vi "LINC Packet Decode.vi"(7 "little endian":bool, 8 "include unit (F)":bool, 9 "binary value (F)":bool, 10 "item formats":T1[](array[typedef]), 11 "data in":string) -> (2 "decoded items":string[](array[string]))   [LabVIEW 2018, in "STEPkgDriver_LINC.lvlib" / "LINC.lvclass"]
uses:
  LINC.lvclass
  STEPkgDriver_LINC.lvlib
  LINC Format Prototype.ctl
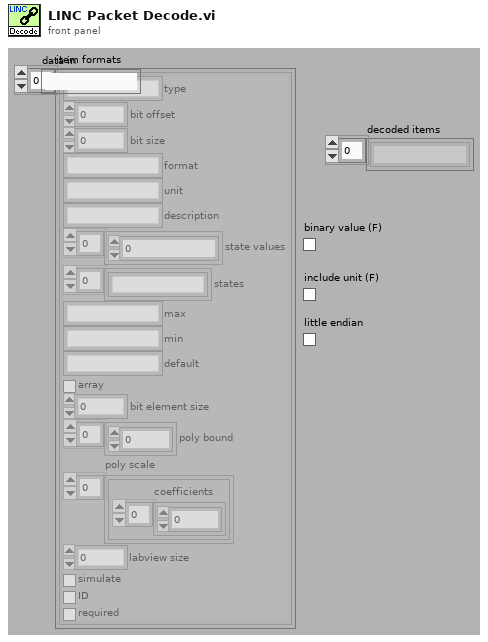
[diagram p1: front panel]
types:
  T1 = typedef "STEPkgDriver_LINC.lvlib/LINC Format Prototype.ctl" = cluster{"type":string, "bit offset":i32, "bit size":i32, "format":string, "unit":string, "description":string, "state values":i64[], "states":string[], "max":string, "min":string, "default":string, "array":bool, "bit element size":i32, "poly bound":dbl[], "poly scale":cluster{"coefficients":dbl[]}[], "labview size":i32, "simulate":bool, "ID":bool, "required":bool}
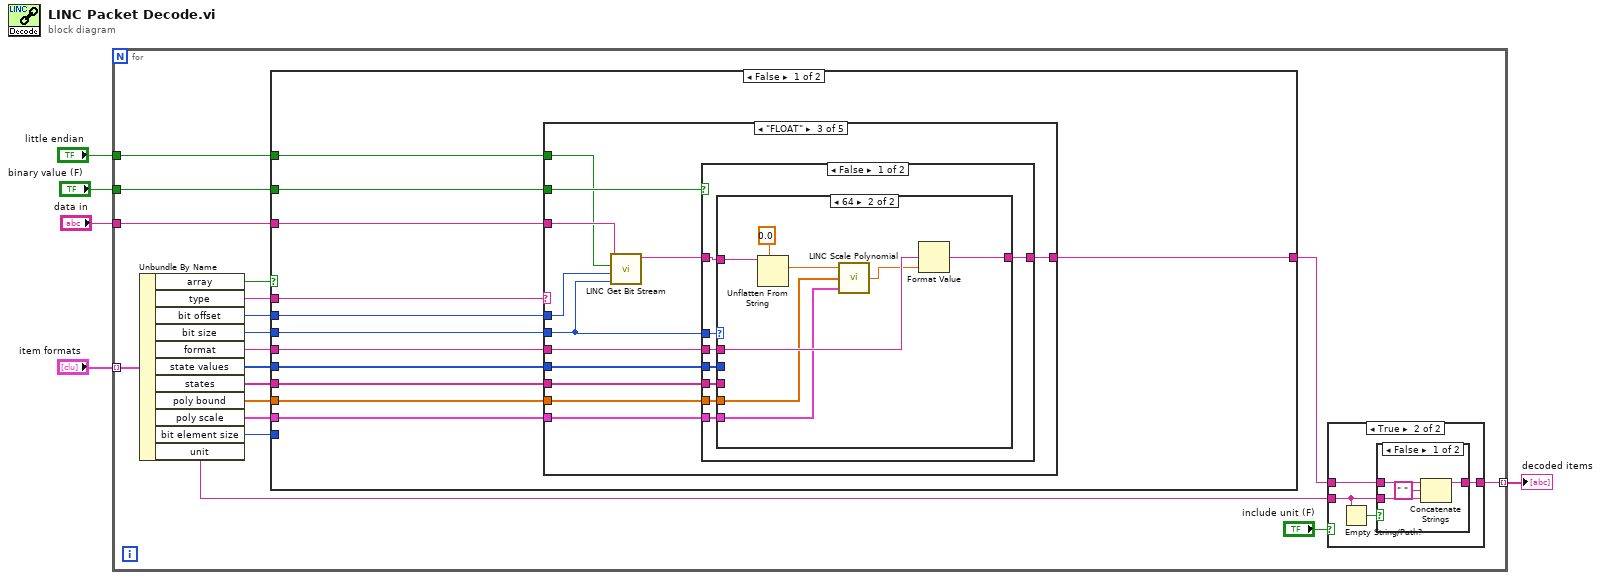
[diagram p0: block diagram]
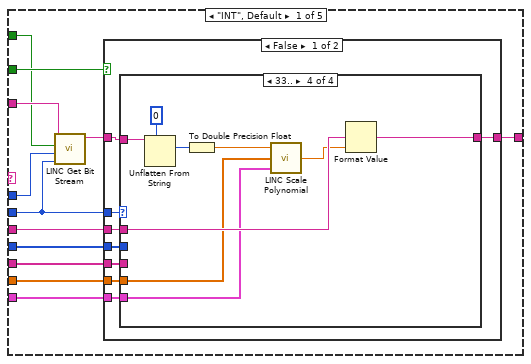
[diagram p2: hidden frame]
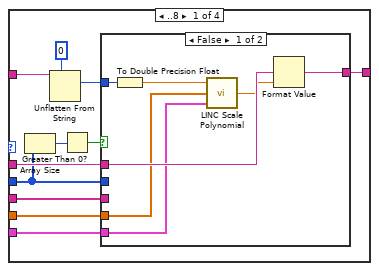
[diagram p3: hidden frame]
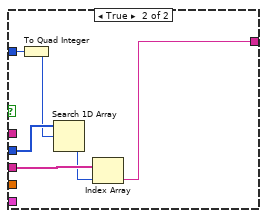
[diagram p4: hidden frame]
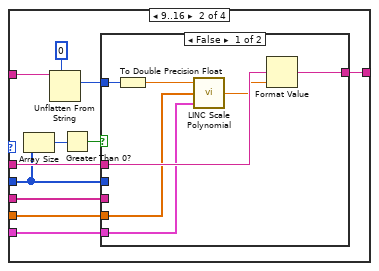
[diagram p5: hidden frame]
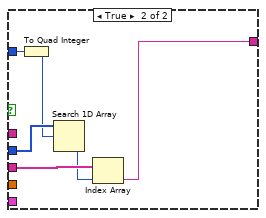
[diagram p6: hidden frame]
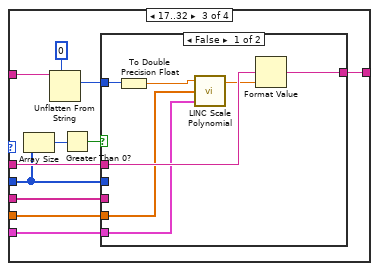
[diagram p7: hidden frame]
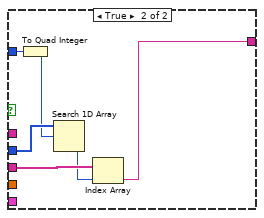
[diagram p8: hidden frame]
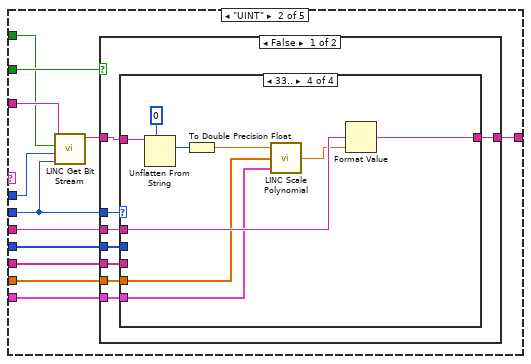
[diagram p10: hidden frame]
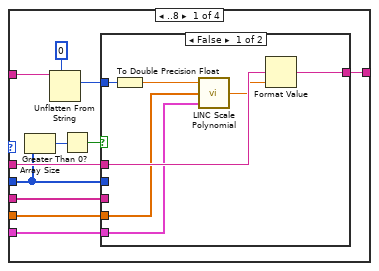
[diagram p11: hidden frame]
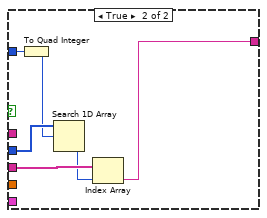
[diagram p12: hidden frame]
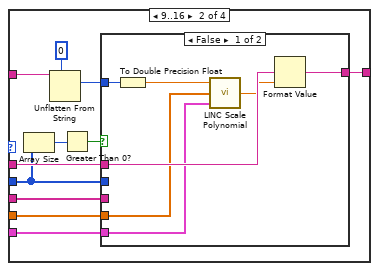
[diagram p13: hidden frame]
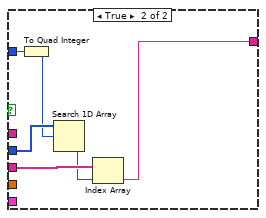
[diagram p14: hidden frame]
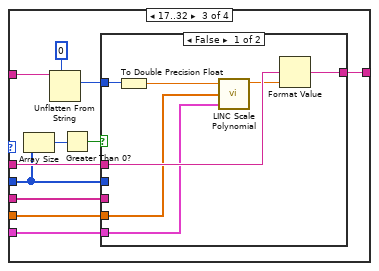
[diagram p15: hidden frame]
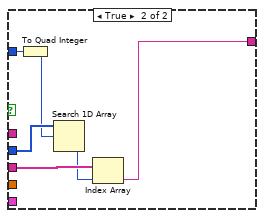
[diagram p16: hidden frame]
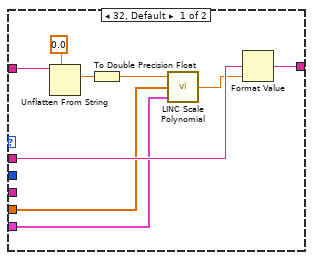
[diagram p18: hidden frame]
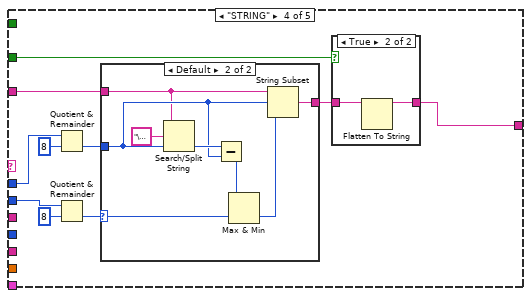
[diagram p20: hidden frame]
diagram:
  n1 = for {
    tunnel: "data in" -> [w13]
    tunnel: "item formats" -> [w23] mode=indexing
    tunnel: [w17] -> w5 mode=indexing
    tunnel: "binary value (F)" -> [w9]
    tunnel: "little endian" -> [w8]
    n2 = Unbundle By Name(w23) -> ("array"=w7:bool, "type"=w22:string, "bit offset"=w14:i32, "bit size"=w15:i32, "format"=w21:string, "state values"=w18:i64[], "states"=w20:string[], "poly bound"=w12:dbl[], "poly scale"=w6:cluster{"coefficients":dbl[]}[], "bit element size"=w16:i32, "unit"=w19:string)
    n3 = case shown="False" w7 {
      tunnel: w22 -> [w35 w342]
      tunnel: w15 -> [w30 w333]
      tunnel: w21 -> [w34 w345]
      tunnel: w20 -> [w33 w343]
      tunnel: [w32 w346] -> w11
      tunnel: w18 -> [w31 w344]
      tunnel: w16 -> [_ w339]
      tunnel: w14 -> [w27 w334]
      tunnel: w12 -> [w29 _]
      tunnel: w13 -> [w28 w335]
      tunnel: w9 -> [w26 w330]
      tunnel: w8 -> [w25 w329]
      tunnel: w6 -> [w24 _]
      frame False {
        n4 = case shown="\"FLOAT\"" w35 {
          tunnel: w30 -> [w43 w141 w241 w282 w306]
          tunnel: [w45 w147 w249 w279 w303] -> w32
          tunnel: w34 -> [w42 w149 w251 _ _]
          tunnel: w33 -> [w40 w148 w250 _ _]
          tunnel: w31 -> [w41 w146 w248 _ _]
          tunnel: w29 -> [w39 w145 w247 _ _]
          tunnel: w28 -> [w47 w144 w245 w284 w308]
          tunnel: w27 -> [w46 w142 w242 w283 w307]
          tunnel: w26 -> [w38 w140 w246 w281 w305]
          tunnel: w25 -> [w37 w139 w243 _ _]
          tunnel: w24 -> [w36 w138 w240 _ _]
          frame "INT", Default {
            n5 = call "LINC Get Bit Stream.vi"("bit size"=w43, "bit offset"=w46, "little endian"=w37, "data in"=w47) -> ("data out"=w44:string)  [unwired: 6 in, 1 out]
            n6 = case shown="False" w38 {
              tunnel: [w55 w137] -> w45
              tunnel: w44 -> [w54 w137]
              tunnel: w43 -> [w53 _]
              tunnel: w42 -> [w52 _]
              tunnel: w41 -> [w51 _]
              tunnel: w40 -> [w50 _]
              tunnel: w39 -> [w49 _]
              tunnel: w36 -> [w48 _]
              frame False {
                n7 = case shown="33.." w53 {
                  tunnel: w54 -> [w66 w90 w114 w136]
                  tunnel: w52 -> [w61 w85 w109 w134]
                  tunnel: w50 -> [w62 w86 w110 _]
                  tunnel: [w59 w83 w107 w133] -> w55
                  tunnel: w51 -> [w58 w82 w106 _]
                  tunnel: w49 -> [w57 w81 w105 w129]
                  tunnel: w48 -> [w56 w80 w104 w128]
                  frame ..8 {
                    n8 = Array Size(array=w58) -> (size(s)=w64:i32)
                    n9 = Unflatten From String(type=i8 0, binary string=w66) -> (value=w60:i8)  [unwired: 3 in, 2 out]
                    n10 = Greater Than 0?(x=w64) -> (x > 0?=w63:bool)
                    n11 = case shown="False" w63 {
                      tunnel: w62 -> [_ w76]
                      tunnel: w61 -> [w73 _]
                      tunnel: w60 -> [w70 w79]
                      tunnel: [w72 w74] -> w59
                      tunnel: w58 -> [_ w78]
                      tunnel: w57 -> [w68 _]
                      tunnel: w56 -> [w67 _]
                      frame False {
                        n12 = To Double Precision Float(number=w70) -> (double precision float=w71:dbl)
                        n13 = call "LINC Scale Polynomial.vi"("poly scale"=w67, "poly bounds"=w68, "unscaled value"=w71) -> ("scaled value"=w69:dbl)
                        n14 = Format Value(format string=w73, value (0)=w69) -> (output string=w72:string)  [unwired: 1 in]
                      }
                      frame True {
                        n15 = To Quad Integer(1:w79) -> (0:w77:i64)
                        n16 = Search 1D Array(1D array=w78, element=w77) -> (index of element=w75:i32)  [unwired: 1 in]
                        n17 = Index Array(array=w76, index=w75) -> (element=w74:string)
                      }
                    }
                  }
                  frame 9..16 {
                    n18 = Array Size(array=w82) -> (size(s)=w88:i32)
                    n19 = Unflatten From String(type=i16 0, binary string=w90) -> (value=w84:i16)  [unwired: 3 in, 2 out]
                    n20 = Greater Than 0?(x=w88) -> (x > 0?=w87:bool)
                    n21 = case shown="False" w87 {
                      tunnel: w86 -> [_ w100]
                      tunnel: w85 -> [w97 _]
                      tunnel: w84 -> [w94 w103]
                      tunnel: [w96 w98] -> w83
                      tunnel: w82 -> [_ w102]
                      tunnel: w81 -> [w92 _]
                      tunnel: w80 -> [w91 _]
                      frame False {
                        n22 = To Double Precision Float(number=w94) -> (double precision float=w95:dbl)
                        n23 = call "LINC Scale Polynomial.vi"("poly scale"=w91, "poly bounds"=w92, "unscaled value"=w95) -> ("scaled value"=w93:dbl)
                        n24 = Format Value(format string=w97, value (0)=w93) -> (output string=w96:string)  [unwired: 1 in]
                      }
                      frame True {
                        n25 = To Quad Integer(1:w103) -> (0:w101:i64)
                        n26 = Search 1D Array(1D array=w102, element=w101) -> (index of element=w99:i32)  [unwired: 1 in]
                        n27 = Index Array(array=w100, index=w99) -> (element=w98:string)
                      }
                    }
                  }
                  frame 17..32 {
                    n28 = Array Size(array=w106) -> (size(s)=w112:i32)
                    n29 = Unflatten From String(type=0, binary string=w114) -> (value=w108:i32)  [unwired: 3 in, 2 out]
                    n30 = Greater Than 0?(x=w112) -> (x > 0?=w111:bool)
                    n31 = case shown="False" w111 {
                      tunnel: w110 -> [_ w124]
                      tunnel: w109 -> [w121 _]
                      tunnel: w108 -> [w118 w127]
                      tunnel: [w120 w122] -> w107
                      tunnel: w106 -> [_ w126]
                      tunnel: w105 -> [w116 _]
                      tunnel: w104 -> [w115 _]
                      frame False {
                        n32 = To Double Precision Float(number=w118) -> (double precision float=w119:dbl)
                        n33 = call "LINC Scale Polynomial.vi"("poly scale"=w115, "poly bounds"=w116, "unscaled value"=w119) -> ("scaled value"=w117:dbl)
                        n34 = Format Value(format string=w121, value (0)=w117) -> (output string=w120:string)  [unwired: 1 in]
                      }
                      frame True {
                        n35 = To Quad Integer(1:w127) -> (0:w125:i64)
                        n36 = Search 1D Array(1D array=w126, element=w125) -> (index of element=w123:i32)  [unwired: 1 in]
                        n37 = Index Array(array=w124, index=w123) -> (element=w122:string)
                      }
                    }
                  }
                  frame 33.. {
                    n38 = Unflatten From String(type=i64 0, binary string=w136) -> (value=w131:i64)  [unwired: 3 in, 2 out]
                    n39 = To Double Precision Float(number=w131) -> (double precision float=w132:dbl)
                    n40 = call "LINC Scale Polynomial.vi"("poly scale"=w128, "poly bounds"=w129, "unscaled value"=w132) -> ("scaled value"=w130:dbl)
                    n41 = Format Value(format string=w134, value (0)=w130) -> (output string=w133:string)  [unwired: 1 in]
                  }
                }
              }
              frame True {
              }
            }
          }
          frame "UINT" {
            n42 = call "LINC Get Bit Stream.vi"("bit size"=w141, "bit offset"=w142, "little endian"=w139, "data in"=w144) -> ("data out"=w143:string)  [unwired: 6 in, 1 out]
            n43 = case shown="False" w140 {
              tunnel: w149 -> [w157 _]
              tunnel: w148 -> [w156 _]
              tunnel: [w155 w239] -> w147
              tunnel: w146 -> [w154 _]
              tunnel: w145 -> [w153 _]
              tunnel: w143 -> [w152 w239]
              tunnel: w141 -> [w151 _]
              tunnel: w138 -> [w150 _]
              frame False {
                n44 = case shown="33.." w151 {
                  tunnel: w152 -> [w168 w192 w216 w238]
                  tunnel: w157 -> [w163 w187 w211 w236]
                  tunnel: w156 -> [w164 w188 w212 _]
                  tunnel: [w161 w185 w209 w235] -> w155
                  tunnel: w154 -> [w160 w184 w208 _]
                  tunnel: w153 -> [w159 w183 w207 w231]
                  tunnel: w150 -> [w158 w182 w206 w230]
                  frame ..8 {
                    n45 = Array Size(array=w160) -> (size(s)=w166:i32)
                    n46 = Unflatten From String(type=u8 0, binary string=w168) -> (value=w162:u8)  [unwired: 3 in, 2 out]
                    n47 = Greater Than 0?(x=w166) -> (x > 0?=w165:bool)
                    n48 = case shown="False" w165 {
                      tunnel: w164 -> [_ w178]
                      tunnel: w163 -> [w175 _]
                      tunnel: w162 -> [w172 w181]
                      tunnel: [w174 w176] -> w161
                      tunnel: w160 -> [_ w180]
                      tunnel: w159 -> [w170 _]
                      tunnel: w158 -> [w169 _]
                      frame False {
                        n49 = To Double Precision Float(number=w172) -> (double precision float=w173:dbl)
                        n50 = call "LINC Scale Polynomial.vi"("poly scale"=w169, "poly bounds"=w170, "unscaled value"=w173) -> ("scaled value"=w171:dbl)
                        n51 = Format Value(format string=w175, value (0)=w171) -> (output string=w174:string)  [unwired: 1 in]
                      }
                      frame True {
                        n52 = To Quad Integer(1:w181) -> (0:w179:i64)
                        n53 = Search 1D Array(1D array=w180, element=w179) -> (index of element=w177:i32)  [unwired: 1 in]
                        n54 = Index Array(array=w178, index=w177) -> (element=w176:string)
                      }
                    }
                  }
                  frame 9..16 {
                    n55 = Array Size(array=w184) -> (size(s)=w190:i32)
                    n56 = Unflatten From String(type=u16 0, binary string=w192) -> (value=w186:u16)  [unwired: 3 in, 2 out]
                    n57 = Greater Than 0?(x=w190) -> (x > 0?=w189:bool)
                    n58 = case shown="False" w189 {
                      tunnel: w188 -> [_ w202]
                      tunnel: w187 -> [w199 _]
                      tunnel: w186 -> [w196 w205]
                      tunnel: [w198 w200] -> w185
                      tunnel: w184 -> [_ w204]
                      tunnel: w183 -> [w194 _]
                      tunnel: w182 -> [w193 _]
                      frame False {
                        n59 = To Double Precision Float(number=w196) -> (double precision float=w197:dbl)
                        n60 = call "LINC Scale Polynomial.vi"("poly scale"=w193, "poly bounds"=w194, "unscaled value"=w197) -> ("scaled value"=w195:dbl)
                        n61 = Format Value(format string=w199, value (0)=w195) -> (output string=w198:string)  [unwired: 1 in]
                      }
                      frame True {
                        n62 = To Quad Integer(1:w205) -> (0:w203:i64)
                        n63 = Search 1D Array(1D array=w204, element=w203) -> (index of element=w201:i32)  [unwired: 1 in]
                        n64 = Index Array(array=w202, index=w201) -> (element=w200:string)
                      }
                    }
                  }
                  frame 17..32 {
                    n65 = Array Size(array=w208) -> (size(s)=w214:i32)
                    n66 = Unflatten From String(type=u32 0, binary string=w216) -> (value=w210:u32)  [unwired: 3 in, 2 out]
                    n67 = Greater Than 0?(x=w214) -> (x > 0?=w213:bool)
                    n68 = case shown="False" w213 {
                      tunnel: w212 -> [_ w226]
                      tunnel: w211 -> [w223 _]
                      tunnel: w210 -> [w220 w229]
                      tunnel: [w222 w224] -> w209
                      tunnel: w208 -> [_ w228]
                      tunnel: w207 -> [w218 _]
                      tunnel: w206 -> [w217 _]
                      frame False {
                        n69 = To Double Precision Float(number=w220) -> (double precision float=w221:dbl)
                        n70 = call "LINC Scale Polynomial.vi"("poly scale"=w217, "poly bounds"=w218, "unscaled value"=w221) -> ("scaled value"=w219:dbl)
                        n71 = Format Value(format string=w223, value (0)=w219) -> (output string=w222:string)  [unwired: 1 in]
                      }
                      frame True {
                        n72 = To Quad Integer(1:w229) -> (0:w227:i64)
                        n73 = Search 1D Array(1D array=w228, element=w227) -> (index of element=w225:i32)  [unwired: 1 in]
                        n74 = Index Array(array=w226, index=w225) -> (element=w224:string)
                      }
                    }
                  }
                  frame 33.. {
                    n75 = Unflatten From String(type=u64 0, binary string=w238) -> (value=w233:u64)  [unwired: 3 in, 2 out]
                    n76 = To Double Precision Float(number=w233) -> (double precision float=w234:dbl)
                    n77 = call "LINC Scale Polynomial.vi"("poly scale"=w230, "poly bounds"=w231, "unscaled value"=w234) -> ("scaled value"=w232:dbl)
                    n78 = Format Value(format string=w236, value (0)=w232) -> (output string=w235:string)  [unwired: 1 in]
                  }
                }
              }
              frame True {
              }
            }
          }
          frame "FLOAT" {
            n79 = call "LINC Get Bit Stream.vi"("bit size"=w241, "bit offset"=w242, "little endian"=w243, "data in"=w245) -> ("data out"=w244:string)  [unwired: 6 in, 1 out]
            n80 = case shown="False" w246 {
              tunnel: w251 -> [w259 _]
              tunnel: w250 -> [w258 _]
              tunnel: [w257 w277] -> w249
              tunnel: w248 -> [w256 _]
              tunnel: w244 -> [w255 w277]
              tunnel: w241 -> [w254 _]
              tunnel: w247 -> [w253 _]
              tunnel: w240 -> [w252 _]
              frame False {
                n81 = case shown="64" w254 {
                  tunnel: w255 -> [w268 w276]
                  tunnel: w259 -> [w266 w274]
                  tunnel: w258 -> [_ _]
                  tunnel: [w265 w273] -> w257
                  tunnel: w256 -> [_ _]
                  tunnel: w253 -> [w261 w270]
                  tunnel: w252 -> [w260 w269]
                  frame 32, Default {
                    n82 = Unflatten From String(type=sgl 0.0, binary string=w268) -> (value=w263:sgl)  [unwired: 3 in, 2 out]
                    n83 = To Double Precision Float(number=w263) -> (double precision float=w264:dbl)
                    n84 = call "LINC Scale Polynomial.vi"("poly scale"=w260, "poly bounds"=w261, "unscaled value"=w264) -> ("scaled value"=w262:dbl)
                    n85 = Format Value(format string=w266, value (0)=w262) -> (output string=w265:string)  [unwired: 1 in]
                  }
                  frame 64 {
                    n86 = Unflatten From String(type=0.0, binary string=w276) -> (value=w272:dbl)  [unwired: 3 in, 2 out]
                    n87 = call "LINC Scale Polynomial.vi"("poly scale"=w269, "poly bounds"=w270, "unscaled value"=w272) -> ("scaled value"=w271:dbl)
                    n88 = Format Value(format string=w274, value (0)=w271) -> (output string=w273:string)  [unwired: 1 in]
                  }
                }
              }
              frame True {
              }
            }
          }
          frame "STRING" {
            n89 = Quotient & Remainder(x=w283, y=8) -> (floor(x/y)=w286:i32)  [unwired: 1 out]
            n90 = Quotient & Remainder(x=w282, y=8) -> (floor(x/y)=w278:i32)  [unwired: 1 out]
            n91 = case shown="Default" w278 {
              selector: w278 -> [_ w291]
              tunnel: w286 -> [w289 w296]
              tunnel: w284 -> [w290 w293]
              tunnel: [w288 w292] -> w280
              frame 0 {
                n92 = String Subset(string=w290, offset (0)=w289) -> (substring=w288:string)  [unwired: 1 in]
              }
              frame Default {
                n93 = Search/Split String(string=w293, search string/char (-)="\u0000", offset (0)=w296) -> (offset of match=w297:i32)  [unwired: 2 out]
                n94 = Subtract(x=w297, y=w296) -> (x-y=w295:i32)
                n95 = Max & Min(x=w295, y=w291) -> (min(x,y)=w294:i32)  [unwired: 1 out]
                n96 = String Subset(string=w293, offset (0)=w296, length (rest)=w294) -> (substring=w292:string)
              }
            }
            n97 = case shown="True" w281 {
              tunnel: w280 -> [w299 w301]
              tunnel: [w299 w300] -> w279
              frame False {
              }
              frame True {
                n98 = Flatten To String(anything=w301) -> (data string=w300:string)  [unwired: 3 in, 2 out]
              }
            }
          }
          frame "BLOCK" {
            n99 = Quotient & Remainder(x=w307, y=8) -> (floor(x/y)=w310:i32)  [unwired: 1 out]
            n100 = Quotient & Remainder(x=w306, y=8) -> (floor(x/y)=w302:i32)  [unwired: 1 out]
            n101 = case shown="0" w302 {
              tunnel: w310 -> [w313 w318]
              tunnel: w308 -> [w314 w317]
              tunnel: [w312 w316] -> w304
              tunnel: w302 -> [_ w315]
              frame 0 {
                n102 = String Subset(string=w314, offset (0)=w313) -> (substring=w312:string)  [unwired: 1 in]
              }
              frame Default {
                n103 = String Subset(string=w317, offset (0)=w318, length (rest)=w315) -> (substring=w316:string)
              }
            }
            n104 = case shown="False" w305 {
              tunnel: w304 -> [w320 w328]
              tunnel: [w319 w327] -> w303
              frame False {
                n105 = String To Byte Array(string=w320) -> (unsigned byte array=w322:u8[])
                n106 = for {
                  tunnel: w322 -> [w326] mode=indexing
                  shift-right: [w324] -> w319
                  shift-left: "" -> [w325]
                  n107 = Format Value(string ("")=w325, format string="%02x", value (0)=w326) -> (output string=w324:string)
                }
              }
              frame True {
                n108 = Flatten To String(anything=w328) -> (data string=w327:string)  [unwired: 3 in, 2 out]
              }
            }
          }
        }
      }
      frame True {
        n109 = Quotient & Remainder(x=w334, y=8) -> (floor(x/y)=w338:i32)  [unwired: 1 out]
        n110 = Quotient & Remainder(x=w333, y=8) -> (floor(x/y)=w331:i32)  [unwired: 1 out]
        n111 = String Subset(string=w335, offset (0)=w338, length (rest)=w331) -> (substring=w332:string)
        n112 = Quotient & Remainder(x=w339, y=8) -> (floor(x/y)=w340:i32)  [unwired: 1 out]
        n113 = case shown="\"INT\", Default" w342 {
          tunnel: w339 -> [w360 w435 w573 _ _]
          tunnel: [w353 w432 w570 w620 w661] -> w346
          tunnel: w345 -> [w359 w434 w572 _ _]
          tunnel: w343 -> [w358 w433 w571 _ _]
          tunnel: w344 -> [w357 w431 w569 _ _]
          tunnel: w340 -> [w348 w422 w560 w617 w658]
          tunnel: w332 -> [w350 w426 w564 w619 w660]
          tunnel: w331 -> [w354 w428 w566 w616 w657]
          tunnel: w330 -> [w352 w427 w565 w615 w656]
          tunnel: w329 -> [w351 w425 w563 _ _]
          frame "INT", Default {
            n114 = Quotient & Remainder(x=w354, y=w348) -> (floor(x/y)=w347:i32)  [unwired: 1 out]
            n115 = case shown="True" w351 {
              tunnel: w350 -> [w361 w365]
              tunnel: [w361 w364] -> w349
              tunnel: w348 -> [_ w362]
              tunnel: w347 -> [_ w363]
              frame False {
              }
              frame True {
                n116 = for {
                  N: w363 -> [_]
                  shift-right: [w369] -> w364
                  shift-left: w365 -> [w370]
                  shift-right: [w373] -> _
                  shift-left: 0 -> [w367]
                  tunnel: w362 -> [w374]
                  tunnel: w362 -> [w372]
                  n117 = String Subset(string=w370, offset (0)=w367, length (rest)=w374) -> (substring=w371:string)
                  n118 = Add(x=w367, y=w372) -> (x+y=w373:i32)
                  n119 = Reverse String(1:w371) -> (0:w368:string)
                  n120 = Replace Substring(3:w367, 4:w368, 5:w370) -> (1:w369:string)  [unwired: 1 in, 1 out]
                }
              }
            }
            n121 = Type Cast(x=w347) -> (*(type *) &x=w355:string)  [unwired: 1 in]
            n122 = Concatenate Strings(w355, w349) -> (w356:string)
            n123 = case shown="False" w352 {
              tunnel: w360 -> [w380 _]
              tunnel: w359 -> [w379 _]
              tunnel: w358 -> [w378 _]
              tunnel: w357 -> [w377 _]
              tunnel: w356 -> [w376 w421]
              tunnel: [w375 w421] -> w353
              frame False {
                n124 = case shown="8, Default" w380 {
                  tunnel: w376 -> [w390 w400 w410 w420]
                  tunnel: w379 -> [w389 w399 w409 w419]
                  tunnel: w378 -> [_ _ _ _]
                  tunnel: [w388 w398 w408 w418] -> w375
                  tunnel: w377 -> [_ _ _ _]
                  frame 8, Default {
                    n125 = Unflatten From String(type=i8[] [], binary string=w390) -> (value=w387:i8[])  [unwired: 3 in, 2 out]
                    n126 = Array To Spreadsheet String(delimiter (Tab)=",", array=w387, 3:w389) -> (spreadsheet string=w382:string)
                    n127 = String Length(string=w382) -> (length=w384:i32)
                    n128 = Subtract(x=w384, y=2) -> (x-y=w381:i32)
                    n129 = String Subset(string=w382, length (rest)=w381) -> (substring=w388:string)  [unwired: 1 in]
                  }
                  frame 16 {
                    n130 = Unflatten From String(type=i16[] [], binary string=w400) -> (value=w397:i16[])  [unwired: 3 in, 2 out]
                    n131 = Array To Spreadsheet String(delimiter (Tab)=",", array=w397, 3:w399) -> (spreadsheet string=w392:string)
                    n132 = String Length(string=w392) -> (length=w394:i32)
                    n133 = Subtract(x=w394, y=2) -> (x-y=w391:i32)
                    n134 = String Subset(string=w392, length (rest)=w391) -> (substring=w398:string)  [unwired: 1 in]
                  }
                  frame 32 {
                    n135 = Unflatten From String(type=i32[] [], binary string=w410) -> (value=w407:i32[])  [unwired: 3 in, 2 out]
                    n136 = Array To Spreadsheet String(delimiter (Tab)=",", array=w407, 3:w409) -> (spreadsheet string=w402:string)
                    n137 = String Length(string=w402) -> (length=w404:i32)
                    n138 = Subtract(x=w404, y=2) -> (x-y=w401:i32)
                    n139 = String Subset(string=w402, length (rest)=w401) -> (substring=w408:string)  [unwired: 1 in]
                  }
                  frame 64 {
                    n140 = Unflatten From String(type=i64[] [], binary string=w420) -> (value=w417:i64[])  [unwired: 3 in, 2 out]
                    n141 = Array To Spreadsheet String(delimiter (Tab)=",", array=w417, 3:w419) -> (spreadsheet string=w412:string)
                    n142 = String Length(string=w412) -> (length=w414:i32)
                    n143 = Subtract(x=w414, y=2) -> (x-y=w411:i32)
                    n144 = String Subset(string=w412, length (rest)=w411) -> (substring=w418:string)  [unwired: 1 in]
                  }
                }
              }
              frame True {
              }
            }
          }
          frame "UINT" {
            n145 = Quotient & Remainder(x=w428, y=w422) -> (floor(x/y)=w423:i32)  [unwired: 1 out]
            n146 = case shown="True" w425 {
              tunnel: w426 -> [w436 w440]
              tunnel: [w436 w439] -> w424
              tunnel: w422 -> [_ w437]
              tunnel: w423 -> [_ w438]
              frame False {
              }
              frame True {
                n147 = for {
                  N: w438 -> [_]
                  shift-right: [w444] -> w439
                  shift-left: w440 -> [w445]
                  shift-right: [w448] -> _
                  shift-left: 0 -> [w442]
                  tunnel: w437 -> [w449]
                  tunnel: w437 -> [w447]
                  n148 = String Subset(string=w445, offset (0)=w442, length (rest)=w449) -> (substring=w446:string)
                  n149 = Add(x=w442, y=w447) -> (x+y=w448:i32)
                  n150 = Reverse String(1:w446) -> (0:w443:string)
                  n151 = Replace Substring(3:w442, 4:w443, 5:w445) -> (1:w444:string)  [unwired: 1 in, 1 out]
                }
              }
            }
            n152 = Type Cast(x=w423) -> (*(type *) &x=w429:string)  [unwired: 1 in]
            n153 = Concatenate Strings(w429, w424) -> (w430:string)
            n154 = case shown="False" w427 {
              tunnel: w435 -> [w455 _]
              tunnel: w434 -> [w454 _]
              tunnel: w433 -> [w453 _]
              tunnel: [w452 w559] -> w432
              tunnel: w431 -> [w451 _]
              tunnel: w430 -> [w450 w559]
              frame False {
                n155 = case shown="8, Default" w455 {
                  tunnel: w450 -> [w464 w495 w526 w558]
                  tunnel: w454 -> [w460 w491 w522 w557]
                  tunnel: w453 -> [w461 w492 w523 _]
                  tunnel: [w458 w489 w520 w555] -> w452
                  tunnel: w451 -> [w457 w488 w519 _]
                  frame 8, Default {
                    n156 = Array Size(array=w457) -> (size(s)=w463:i32)
                    n157 = Unflatten From String(type=u8[] [], binary string=w464) -> (value=w459:u8[])  [unwired: 3 in, 2 out]
                    n158 = Greater Than 0?(x=w463) -> (x > 0?=w462:bool)
                    n159 = case shown="True" w462 {
                      tunnel: w461 -> [_ w476]
                      tunnel: w460 -> [w472 _]
                      tunnel: w459 -> [w471 w478]
                      tunnel: [w465 w473] -> w458
                      tunnel: w457 -> [_ w477]
                      frame False {
                        n160 = Array To Spreadsheet String(delimiter (Tab)=",", array=w471, 3:w472) -> (spreadsheet string=w467:string)
                        n161 = String Length(string=w467) -> (length=w469:i32)
                        n162 = Subtract(x=w469, y=2) -> (x-y=w466:i32)
                        n163 = String Subset(string=w467, length (rest)=w466) -> (substring=w465:string)  [unwired: 1 in]
                      }
                      frame True {
                        n164 = To Unsigned Long Integer(number=w478) -> (unsigned 32bit integer=w475:u32[])
                        n165 = for {
                          tunnel: w477 -> [w486]
                          tunnel: w476 -> [w485]
                          tunnel: w475 -> [w483] mode=indexing
                          shift-right: [w481] -> _
                          shift-left: "" -> [w479]
                          tunnel: [w479] -> w473
                          n166 = Search 1D Array(1D array=w486, element=w483) -> (index of element=w484:i32)  [unwired: 1 in]
                          n167 = Index Array(array=w485, index=w484) -> (element=w482:string)
                          n168 = Concatenate Strings(w479, w482, ",") -> (w481:string)
                        }
                      }
                    }
                  }
                  frame 16 {
                    n169 = Array Size(array=w488) -> (size(s)=w494:i32)
                    n170 = Unflatten From String(type=u16[] [], binary string=w495) -> (value=w490:u16[])  [unwired: 3 in, 2 out]
                    n171 = Greater Than 0?(x=w494) -> (x > 0?=w493:bool)
                    n172 = case shown="True" w493 {
                      tunnel: w492 -> [_ w507]
                      tunnel: w491 -> [w503 _]
                      tunnel: w490 -> [w502 w509]
                      tunnel: [w496 w504] -> w489
                      tunnel: w488 -> [_ w508]
                      frame False {
                        n173 = Array To Spreadsheet String(delimiter (Tab)=",", array=w502, 3:w503) -> (spreadsheet string=w498:string)
                        n174 = String Length(string=w498) -> (length=w500:i32)
                        n175 = Subtract(x=w500, y=2) -> (x-y=w497:i32)
                        n176 = String Subset(string=w498, length (rest)=w497) -> (substring=w496:string)  [unwired: 1 in]
                      }
                      frame True {
                        n177 = To Unsigned Long Integer(number=w509) -> (unsigned 32bit integer=w506:u32[])
                        n178 = for {
                          tunnel: w508 -> [w517]
                          tunnel: w507 -> [w516]
                          tunnel: w506 -> [w514] mode=indexing
                          shift-right: [w512] -> _
                          shift-left: "" -> [w510]
                          tunnel: [w510] -> w504
                          n179 = Search 1D Array(1D array=w517, element=w514) -> (index of element=w515:i32)  [unwired: 1 in]
                          n180 = Index Array(array=w516, index=w515) -> (element=w513:string)
                          n181 = Concatenate Strings(w510, w513, ",") -> (w512:string)
                        }
                      }
                    }
                  }
                  frame 32 {
                    n182 = Array Size(array=w519) -> (size(s)=w525:i32)
                    n183 = Unflatten From String(type=u32[] [], binary string=w526) -> (value=w521:u32[])  [unwired: 3 in, 2 out]
                    n184 = Greater Than 0?(x=w525) -> (x > 0?=w524:bool)
                    n185 = case shown="True" w524 {
                      tunnel: w523 -> [_ w538]
                      tunnel: w522 -> [w534 _]
                      tunnel: w521 -> [w533 w540]
                      tunnel: [w527 w535] -> w520
                      tunnel: w519 -> [_ w539]
                      frame False {
                        n186 = Array To Spreadsheet String(delimiter (Tab)=",", array=w533, 3:w534) -> (spreadsheet string=w529:string)
                        n187 = String Length(string=w529) -> (length=w531:i32)
                        n188 = Subtract(x=w531, y=2) -> (x-y=w528:i32)
                        n189 = String Subset(string=w529, length (rest)=w528) -> (substring=w527:string)  [unwired: 1 in]
                      }
                      frame True {
                        n190 = To Unsigned Long Integer(number=w540) -> (unsigned 32bit integer=w537:u32[])
                        n191 = for {
                          tunnel: w539 -> [w548]
                          tunnel: w538 -> [w547]
                          tunnel: w537 -> [w545] mode=indexing
                          shift-right: [w543] -> _
                          shift-left: "" -> [w541]
                          tunnel: [w541] -> w535
                          n192 = Search 1D Array(1D array=w548, element=w545) -> (index of element=w546:i32)  [unwired: 1 in]
                          n193 = Index Array(array=w547, index=w546) -> (element=w544:string)
                          n194 = Concatenate Strings(w541, w544, ",") -> (w543:string)
                        }
                      }
                    }
                  }
                  frame 64 {
                    n195 = Unflatten From String(type=u64[] [], binary string=w558) -> (value=w556:u64[])  [unwired: 3 in, 2 out]
                    n196 = Array To Spreadsheet String(delimiter (Tab)=",", array=w556, 3:w557) -> (spreadsheet string=w550:string)
                    n197 = String Length(string=w550) -> (length=w552:i32)
                    n198 = Subtract(x=w552, y=2) -> (x-y=w549:i32)
                    n199 = String Subset(string=w550, length (rest)=w549) -> (substring=w555:string)  [unwired: 1 in]
                  }
                }
              }
              frame True {
              }
            }
          }
          frame "FLOAT" {
            n200 = Quotient & Remainder(x=w566, y=w560) -> (floor(x/y)=w561:i32)  [unwired: 1 out]
            n201 = case shown="True" w563 {
              tunnel: w564 -> [w574 w578]
              tunnel: [w574 w577] -> w562
              tunnel: w560 -> [_ w575]
              tunnel: w561 -> [_ w576]
              frame False {
              }
              frame True {
                n202 = for {
                  N: w576 -> [_]
                  shift-right: [w582] -> w577
                  shift-left: w578 -> [w583]
                  shift-right: [w586] -> _
                  shift-left: 0 -> [w580]
                  tunnel: w575 -> [w587]
                  tunnel: w575 -> [w585]
                  n203 = String Subset(string=w583, offset (0)=w580, length (rest)=w587) -> (substring=w584:string)
                  n204 = Add(x=w580, y=w585) -> (x+y=w586:i32)
                  n205 = Reverse String(1:w584) -> (0:w581:string)
                  n206 = Replace Substring(3:w580, 4:w581, 5:w583) -> (1:w582:string)  [unwired: 1 in, 1 out]
                }
              }
            }
            n207 = Type Cast(x=w561) -> (*(type *) &x=w567:string)  [unwired: 1 in]
            n208 = Concatenate Strings(w567, w562) -> (w568:string)
            n209 = case shown="False" w565 {
              tunnel: w573 -> [w593 _]
              tunnel: w572 -> [w592 _]
              tunnel: w571 -> [w591 _]
              tunnel: [w590 w614] -> w570
              tunnel: w569 -> [w589 _]
              tunnel: w568 -> [w588 w614]
              frame False {
                n210 = case shown="32, Default" w593 {
                  tunnel: w588 -> [w603 w613]
                  tunnel: w592 -> [w602 w612]
                  tunnel: w591 -> [_ _]
                  tunnel: [w600 w610] -> w590
                  tunnel: w589 -> [_ _]
                  frame 32, Default {
                    n211 = Unflatten From String(type=sgl[] [], binary string=w603) -> (value=w601:sgl[])  [unwired: 3 in, 2 out]
                    n212 = Array To Spreadsheet String(delimiter (Tab)=",", array=w601, 3:w602) -> (spreadsheet string=w595:string)
                    n213 = String Length(string=w595) -> (length=w597:i32)
                    n214 = Subtract(x=w597, y=2) -> (x-y=w594:i32)
                    n215 = String Subset(string=w595, length (rest)=w594) -> (substring=w600:string)  [unwired: 1 in]
                  }
                  frame 64 {
                    n216 = Unflatten From String(type=dbl[] [], binary string=w613) -> (value=w611:dbl[])  [unwired: 3 in, 2 out]
                    n217 = Array To Spreadsheet String(delimiter (Tab)=",", array=w611, 3:w612) -> (spreadsheet string=w605:string)
                    n218 = String Length(string=w605) -> (length=w607:i32)
                    n219 = Subtract(x=w607, y=2) -> (x-y=w604:i32)
                    n220 = String Subset(string=w605, length (rest)=w604) -> (substring=w610:string)  [unwired: 1 in]
                  }
                }
              }
              frame True {
              }
            }
          }
          frame "STRING" {
            n221 = Quotient & Remainder(x=w616, y=w617) -> (floor(x/y)=w618:i32)  [unwired: 1 out]
            n222 = case shown="True" w615 {
              tunnel: [w624 w638] -> w620
              tunnel: w619 -> [w623 w642]
              tunnel: w618 -> [w622 w641]
              tunnel: w617 -> [w621 w643]
              frame False {
                n223 = for {
                  N: w622 -> [_]
                  tunnel: w621 -> [w634]
                  tunnel: w623 -> [w637]
                  shift-right: [w635] -> _
                  shift-left: 0 -> [w636]
                  shift-right: [w628] -> _
                  shift-left: "" -> [w630]
                  tunnel: [w627] -> w624
                  n224 = String Subset(string=w637, offset (0)=w636, length (rest)=w634) -> (substring=w632:string)
                  n225 = Add(x=w636, y=w634) -> (x+y=w635:i32)
                  n226 = Search/Split String(string=w632, search string/char (-)="\u0000") -> (substring before match=w631:string)  [unwired: 3 out]
                  n227 = Concatenate Strings(w630, w631) -> (w627:string)
                  n228 = Concatenate Strings(w627, ",") -> (w628:string)
                }
              }
              frame True {
                n229 = for {
                  N: w641 -> [_]
                  tunnel: w643 -> [w652]
                  tunnel: w642 -> [w655]
                  shift-right: [w653] -> _
                  shift-left: 0 -> [w654]
                  shift-right: [w648] -> w640
                  shift-left: "" -> [w649]
                  n230 = String Subset(string=w655, offset (0)=w654, length (rest)=w652) -> (substring=w650:string)
                  n231 = Add(x=w654, y=w652) -> (x+y=w653:i32)
                  n232 = Search/Split String(string=w650, search string/char (-)="\u0000") -> (substring before match=w647:string)  [unwired: 3 out]
                  n233 = Flatten To String(anything=w647) -> (data string=w646:string)  [unwired: 3 in, 2 out]
                  n234 = Concatenate Strings(w649, w646) -> (w648:string)
                }
                n235 = Type Cast(x=w641) -> (*(type *) &x=w639:string)  [unwired: 1 in]
                n236 = Concatenate Strings(w639, w640) -> (w638:string)
              }
            }
          }
          frame "BLOCK" {
            n237 = Quotient & Remainder(x=w657, y=w658) -> (floor(x/y)=w659:i32)  [unwired: 1 out]
            n238 = case shown="False" w656 {
              tunnel: [w665 w684] -> w661
              tunnel: w660 -> [w664 w688]
              tunnel: w659 -> [w663 w687]
              tunnel: w658 -> [w662 w689]
              frame False {
                n239 = for {
                  N: w663 -> [_]
                  tunnel: w662 -> [w676]
                  tunnel: w664 -> [w679]
                  shift-right: [w677] -> _
                  shift-left: 0 -> [w678]
                  shift-right: [w673] -> _
                  shift-left: "" -> [w675]
                  tunnel: [w672] -> w665
                  n240 = String Subset(string=w679, offset (0)=w678, length (rest)=w676) -> (substring=w669:string)
                  n241 = Add(x=w678, y=w676) -> (x+y=w677:i32)
                  n242 = String To Byte Array(string=w669) -> (unsigned byte array=w671:u8[])
                  n243 = for {
                    tunnel: w671 -> [w683] mode=indexing
                    shift-right: [w681] -> w668
                    shift-left: "" -> [w682]
                    n244 = Format Value(string ("")=w682, format string="%02x", value (0)=w683) -> (output string=w681:string)
                  }
                  n245 = Concatenate Strings(w675, w668) -> (w672:string)
                  n246 = Concatenate Strings(w672, ",") -> (w673:string)
                }
              }
              frame True {
                n247 = for {
                  N: w687 -> [_]
                  tunnel: w689 -> [w696]
                  tunnel: w688 -> [w699]
                  shift-right: [w697] -> _
                  shift-left: 0 -> [w698]
                  shift-right: [w694] -> w686
                  shift-left: "" -> [w695]
                  n248 = String Subset(string=w699, offset (0)=w698, length (rest)=w696) -> (substring=w692:string)
                  n249 = Add(x=w698, y=w696) -> (x+y=w697:i32)
                  n250 = Flatten To String(anything=w692) -> (data string=w693:string)  [unwired: 3 in, 2 out]
                  n251 = Concatenate Strings(w695, w693) -> (w694:string)
                }
                n252 = Type Cast(x=w687) -> (*(type *) &x=w685:string)  [unwired: 1 in]
                n253 = Concatenate Strings(w685, w686) -> (w684:string)
              }
            }
          }
        }
      }
    }
    n254 = case shown="True" "include unit (F)" {
      tunnel: w11 -> [w700 w704]
      tunnel: w19 -> [_ w702]
      tunnel: [w700 w703] -> w17
      frame False {
      }
      frame True {
        n255 = Empty String/Path?(string/path=w702) -> (empty?=w701:bool)
        n256 = case shown="False" w701 {
          tunnel: w704 -> [w708 w709]
          tunnel: [w706 w709] -> w703
          tunnel: w702 -> [w705 _]
          frame False {
            n257 = Concatenate Strings(w708, " " ("string"), w705) -> (w706:string)
          }
          frame True {
          }
        }
      }
    }
  }
  "decoded items" <- w5
